vi "Slope.vi"(1 "Y2":dbl, 2 "X2":dbl, 3 "Y1":dbl, 4 "X1":dbl) -> (0 "SLOPE":dbl)   [LabVIEW 2020]
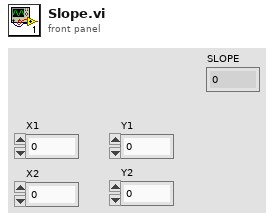
[diagram p1: front panel]
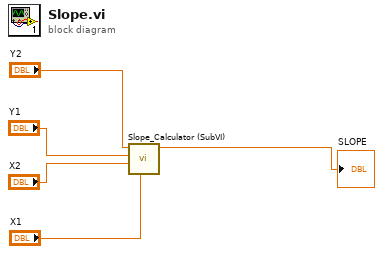
[diagram p0: block diagram]
diagram:
  n1 = call "Slope_Calculator (SubVI).vi"("X1"="X1", "X2"="X2", "Y1"="Y1", "Y2"="Y2") -> ("Numeric"=→"SLOPE":dbl)  [unwired: 7 in]
